vi "Drive Base Immediate.vi"(7 "Operation":T2, 8 "Command Info In":T3, 9 "Path Planner Data":T1, 10 "Right Setpoint":dbl, 11 "Left Setpoint":dbl) -> (0 "Command Info Out":T3)   [LabVIEW 2019]
doc: "This template includes code for deadband comparision to avoid excessive command scheduling. It is particularly useful for joystick-driven commands.\n\nBe sure to right-click and select New from Template and save with a new command name."
uses:
  <vilib>/Rock Robotics/WPI/Framework/Command Status Info.ctl
  <vilib>/Rock Robotics/WPI/Framework/Completion Status.ctl
  <vilib>/Rock Robotics/WPI/Framework/Completion Notifier.ctl
  Implementation/Drive Base Operations.ctl
  Path Planner Data.ctl
  Implementation/Drive Base Setpoints.ctl
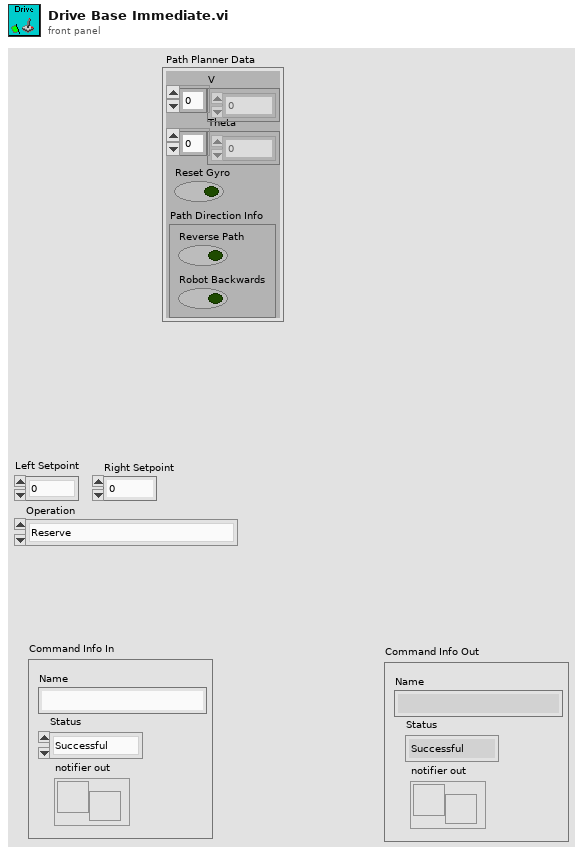
[diagram p1: front panel]
types:
  T1 = typedef "Path Planner Data.ctl" = cluster{"Reset Gyro":bool, "Path Direction Info":cluster{"Reverse Path":bool, "Robot Backwards":bool}, "Theta":dbl[], "V":dbl[]}
  T2 = typedef "Drive Base Operations.ctl" = enum16{"Reserve", "Read Current", "Immediate", "Limelight", "Manual Adjustment", "Limelight + Shoot", "Play Path"}
  T3 = typedef "Command Status Info.ctl" = cluster{"Name":string, "Status":T4, "notifier out":T5}
  T4 = typedef "Completion Status.ctl" = enum16{"Successful", "Aborted", "Incomplete"}
  T5 = typedef "Completion Notifier.ctl" = refnum<notifier>
  T6 = typedef "Drive Base Setpoints.ctl" = cluster{"Operation":T2, "Left Setpoint":dbl, "Duration":dbl, "Right Setpoint":dbl, "Path Planner Data":T1, "Command Sequencer Info":cluster{"Time (s)":dbl, "Name":string, "All Control Values Variant":cluster{"Name":string, "Variant Data":variant}[]}[]}
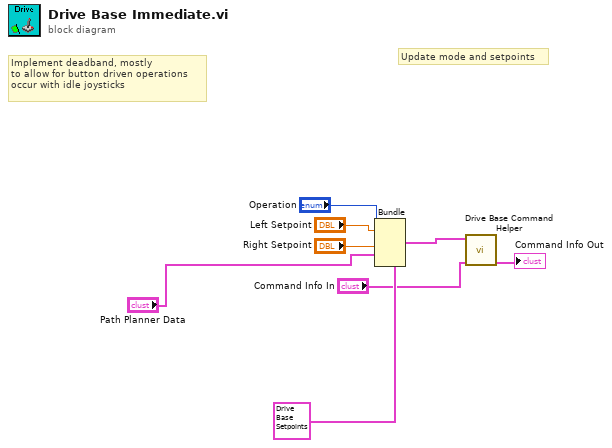
[diagram p0: block diagram]
diagram:
  # "Implement deadband, mostly\nto allow for button driven operations\noccur with idle joysticks"
  # "Update mode and setpoints"
  n1 = Bundle(cluster=T6 {"Operation"=enum."Immediate", "Left Setpoint"=0.0, "Duration"=0.0, "Right Setpoint"=0.0, "Path Planner Data"={"Reset Gyro"=FALSE, "Path Direction Info"={"Reverse Path"=FALSE, "Robot Backwards"=FALSE}, "Theta"=[], "V"=[]}, "Command Sequencer Info"=[]} ("SubSystem Data"), "Operation"="Operation", "Left Setpoint"="Left Setpoint", "Right Setpoint"="Right Setpoint", "Path Planner Data"="Path Planner Data") -> (w7:T6)  [unwired: 2 in]
  n2 = call "Drive Base Command Helper.vi"("Command Info In"="Command Info In", "SubSystem Data"=w7) -> ("Command Info Out"=→"Command Info Out":T3)  [unwired: 7 in, 2 out]
